vi "write_bytes.vi"(8 "error in (no error)":errorcluster, 9 "timeout ms (-1)":i32=-1, 10 "data in":string, 11 "Connection in":refnum<class "Connection.lvclass">) -> (0 "error out":errorcluster, 1 "bytes written":i32, 2 "timeout?":bool, 3 "Connection out":refnum<class "Connection.lvclass">)   [LabVIEW 2019, in "Socket API.lvlib" / "Connection.lvclass"]
uses:
  Connection.lvclass
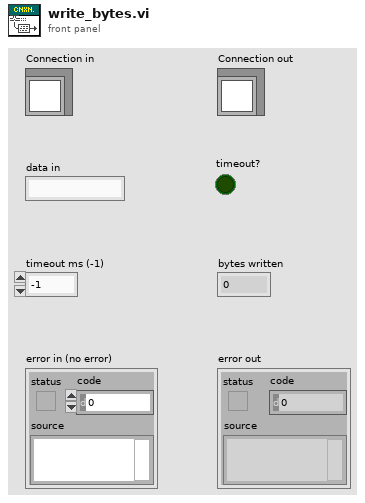
[diagram p1: front panel]
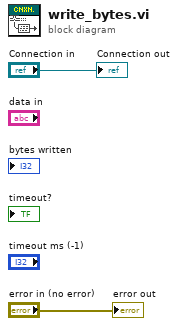
[diagram p0: block diagram]
diagram:
  "error out" <- "error in (no error)"
  "Connection out" <- "Connection in"
